vi "Count by Status.vi"(10 "Status":T1, 11 "Test Case Result In":refnum<class "Test Case Result.lvclass">) -> (2 "Count":i32, 3 "Test Case Result Out":refnum<class "Test Case Result.lvclass">)   [LabVIEW 2020, in "Test Case Result.lvclass"]
uses:
  Test Case Result.lvclass
  Assertion Result/Public/TypeDefs/Status.ctl
  Test Case Result.lvclass/Test Case Result.ctl
  Method Result/Method Result.lvclass/Method Result.ctl
  Method Result/Method Result.lvclass
  Assertion Result/Assertion Result.lvclass
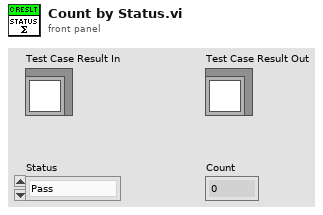
[diagram p1: front panel]
types:
  T1 = typedef "Assertion Result.lvclass/Status.ctl" = enum16{"Pass", "Fail", "Error", "Skipped", "Setup Error", "Broken", "Teardown Error"}
  T2 = map{string, refnum<class "Method Result.lvclass">}
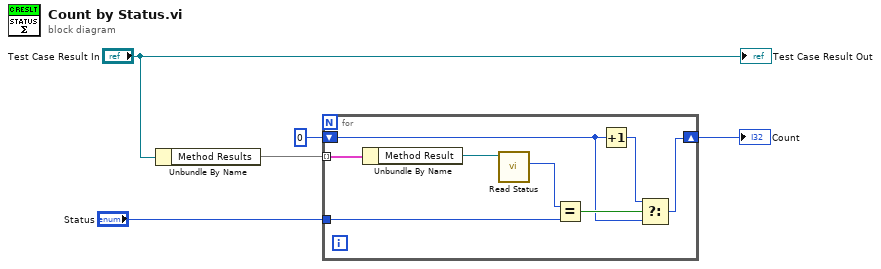
[diagram p0: block diagram]
diagram:
  n1 = Unbundle By Name("Test Case Result In") -> ("Method Results"=w4:T2)
  n2 = for {
    tunnel: w4 -> [w6] mode=indexing
    shift-right: [w9] -> w3
    shift-left: 0 -> [w10]
    tunnel: "Status" -> [w8]
    n3 = Unbundle By Name(w6) -> ("Method Result"=w7:refnum<class "Method Result.lvclass">)
    n4 = call "Read Status.vi"("Method Result In"=w7) -> ("Status"=w13:T1)  [unwired: 8 in, 2 out]
    n5 = Equal?(x=w13, y=w8) -> (x = y?=w12:bool)
    n6 = Increment(x=w10) -> (x+1=w11:i32)
    n7 = Select(t=w11, s=w12, f=w10) -> (s? t:f=w9:i32)
  }
  "Count" <- w3
  "Test Case Result Out" <- "Test Case Result In"
